vi "Read Finished.vi"(8 "error in (no error)":errorcluster, 11 "Scheduile Array in":refnum<class "Scheduile Array.lvclass">) -> (0 "error out":errorcluster, 2 "Finished":bool, 3 "Scheduile Array out":refnum<class "Scheduile Array.lvclass">)   [LabVIEW 2015, in "Scheduile Array.lvclass"]
uses:
  Scheduile Array.lvclass
  Schedule.lvclass
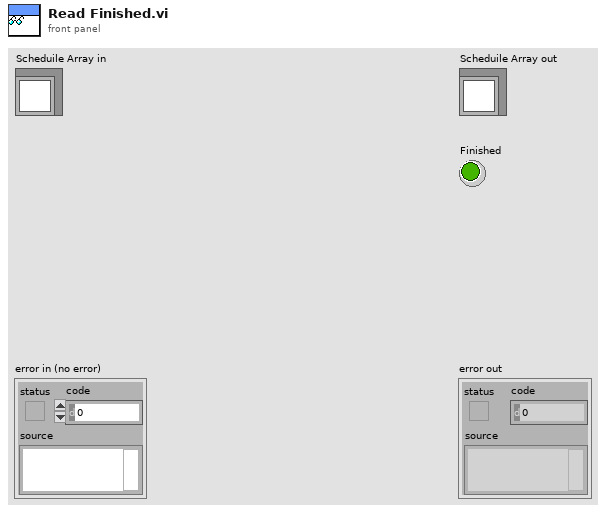
[diagram p1: front panel]
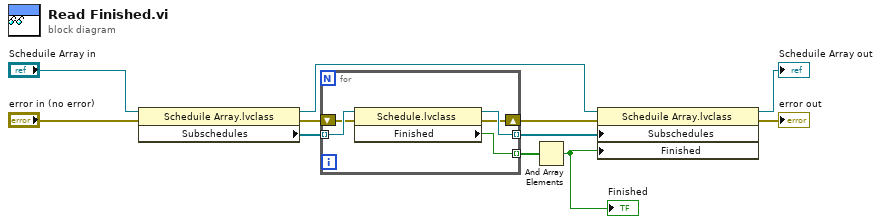
[diagram p0: block diagram]
diagram:
  n1 = property class="Scheduile Array.lvclass"(reference="Scheduile Array in", error in="error in (no error)") -> (reference out=w8:refnum<class "Scheduile Array.lvclass">, error out=w7:errorcluster, "Subschedules"=w10:refnum<class "Schedule.lvclass">[])
  n2 = for {
    tunnel: w10 -> [w16] mode=indexing
    tunnel: [w15] -> w5 mode=indexing
    tunnel: [w14] -> w9 mode=indexing
    shift-right: [w12] -> w6
    shift-left: w7 -> [w13]
    n3 = property class="Schedule.lvclass"(reference=w16, error in=w13) -> (reference out=w14:refnum<class "Schedule.lvclass">, error out=w12:errorcluster, "Finished"=w15:bool)
  }
  n4 = And Array Elements(Boolean array=w5) -> (logical AND=w1:bool)
  "Finished" <- w1
  n5 = property class="Scheduile Array.lvclass"(reference=w8, error in=w6, "Subschedules"=w9, "Finished"=w1) -> (reference out=→"Scheduile Array out":refnum<class "Scheduile Array.lvclass">, error out=→"error out":errorcluster)
